vi "主控件位置移动.vi"(9 "全局坐标":T2 caption="坐标 全局变量", 10 "目标坐标":T1={"Left"=-2000, "Top"=870}, 11 "引用":refnum<vi>) -> (3 "目标位置":T1={"Left"=-2000, "Top"=870} caption="目标坐标")   [LabVIEW 2015]
uses:
  <vilib>/Utility/miscctls.llb/LVPoint32TypeDef.ctl
  <vilib>/Utility/miscctls.llb/LVPositionTypeDef.ctl
panel:
  out "x-y":i32
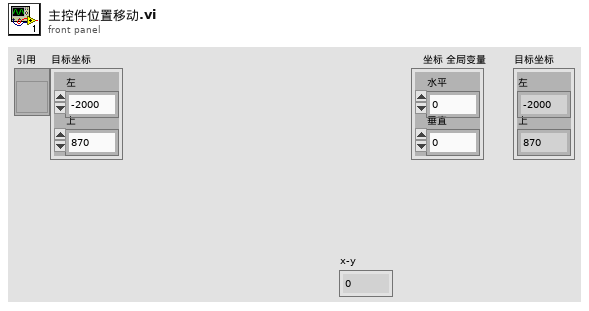
[diagram p1: front panel]
types:
  T1 = typedef "LVPositionTypeDef.ctl" = cluster{"Left":i32, "Top":i32}
  T2 = typedef "LVPoint32TypeDef.ctl" = cluster{"Horizontal":i32, "Vertical":i32}
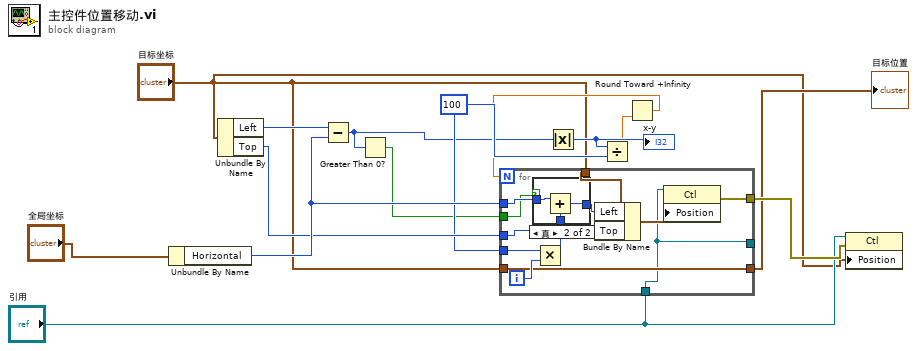
[diagram p0: block diagram]
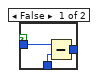
[diagram p2: hidden frame]
diagram:
  w10 = 100 ("y")
  n1 = Unbundle By Name("全局坐标") -> ("Horizontal"=w13:i32)
  n2 = Unbundle By Name("目标坐标") -> ("Left"=w14:i32, "Top"=w12:i32)
  n3 = Subtract(x=w14, y=w13) -> (x-y=w2:i32)
  n4 = Greater Than 0?(x=w2) -> (x > 0?=w1:bool)
  n5 = Absolute Value(x=w2) -> (abs(x)=w11:i32)
  "x-y" <- w11
  n6 = Divide(x=w11, y=w10) -> (x/y=w9:dbl)
  n7 = Round Toward +Infinity(x=w9) -> (ceil(x): smallest int >= x=w8:dbl)
  n8 = for {
    N: w8 -> [_]
    tunnel: w13 -> [w26]
    tunnel: "目标坐标" -> [w25]
    tunnel: w12 -> [w23]
    tunnel: w10 -> [w21]
    tunnel: "目标坐标" -> [w18]
    tunnel: [w18] -> w5
    tunnel: "引用" -> [w17]
    tunnel: [w17] -> _
    tunnel: [w16] -> w6
    tunnel: w1 -> [w15]
    i -> [w20]
    n9 = Multiply(x=w21, y=w20) -> (x*y=w19:i32)
    n10 = case shown="真" w15 {
      tunnel: w26 -> [w29 w31]
      tunnel: [w28 w30] -> w24
      tunnel: w19 -> [w27 w32]
      frame False {
        n11 = Subtract(x=w29, y=w27) -> (x-y=w28:i32)
      }
      frame True {
        n12 = Add(x=w31, y=w32) -> (x+y=w30:i32)
      }
    }
    n13 = Bundle By Name(cluster=w25, "Left"=w24, "Top"=w23) -> (w22:T1)
    n14 = property on="属性节点" class="Ctl"(reference=w17, "Position"=w22) -> (error out=w16:errorcluster)  [unwired: 1 in, 1 out]
  }
  "目标位置" <- w5
  n15 = property on="属性节点" class="Ctl"(reference="引用", error in=w6, "Position"="目标坐标") -> ()  [unwired: 2 out]
